vi "KE622x -- Turn Output On And Check For Errors.vi"(0 "Resource In":refnum<visa-resource-name>, 1 "Check For SCPI Errors? (T)":bool=TRUE, 5 "Turn Off Output If Compliance?":bool=TRUE, 11 "error in (no error)":errorcluster, 12 "Compliance Check Delay (500 ms)":u32=500) -> (4 "Resource Out (dupl)":refnum<visa-resource-name>, 6 "Interlock Tripped?":bool, 8 "Compliance?":bool, 15 "error out":errorcluster)   [LabVIEW 2013, in "Keithly user program.lvlib"]
uses:
  Keithly user program.lvlib
  Typedefs/KE622x -- On Off Control.ctl
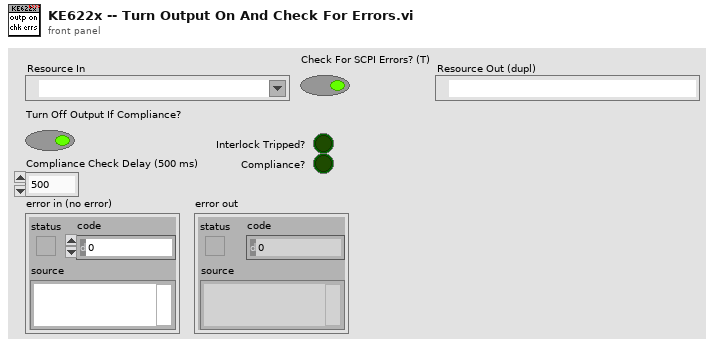
[diagram p1: front panel]
types:
  T1 = typedef "Keithly user program.lvlib/KE622x -- On Off Control.ctl" = enum16{"Off", "On"}
  T2 = typedef "Keithly user program.lvlib/KE622x -- Meas Event Reg State.ctl" = cluster{"B0, ROF:  KE2182A Delta Reading Overflow Event?":bool, "B1, Int:  Interlock OK Event?":bool, "B2, Temp:  Over Temperature Event?":bool, "B3, Comp:  Compliance Event?":bool, "B5, RAV:  Delta Reading Available Event?":bool, "B6, TN:  User Defined Reading Number Stored In Buffer Event?":bool, "B7, BAV:  At Least 2 Readings Stored In Buffer Event?":bool, "B12, BQF:  Buffer Quarter Full Event?":bool, "B8, BHF:  Buffer Half Full Event?":bool, "B13, B3QF:  Buffer 3/4 Full Event?":bool, "B9, BFL:  Buffer Full Event?":bool}
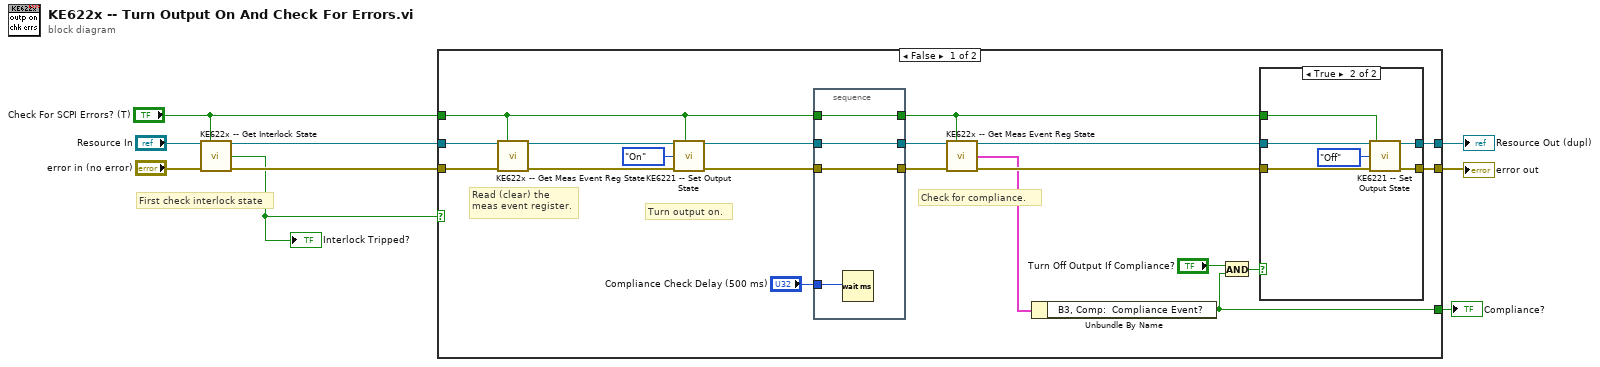
[diagram p0: block diagram]
diagram:
  # "First check interlock state"
  n1 = call "KE622x -- Get Interlock State.vi"("Resource In"="Resource In", "Check For SCPI Errors? (T)"="Check For SCPI Errors? (T)", "error in (no error)"="error in (no error)") -> ("Resource Out (dupl)"=w6:refnum<visa-resource-name>, "Interlock Tripped?"=w2:bool, "error out"=w3:errorcluster)  [unwired: 10 in]
  "Interlock Tripped?" <- w2
  n2 = case shown="False" w2 {
    tunnel: w3 -> [w22 w42]
    tunnel: w6 -> [w23 w43]
    tunnel: "Check For SCPI Errors? (T)" -> [w20 _]
    tunnel: [w27 _] -> w9
    tunnel: [w25 w42] -> w7
    tunnel: [w24 w43] -> w8
    frame False {
      # "Read (clear) the\nmeas event register."
      # "Turn output on."
      # "Check for compliance."
      n3 = call "KE622x -- Get Meas Event Reg State.vi"("VISA Resource In"=w23, "Error Query (T)?"=w20, "error in (no error)"=w22) -> ("VISA Resource Out (dupl)"=w19:refnum<visa-resource-name>, "error out"=w18:errorcluster)  [unwired: 10 in, 1 out]
      n4 = call "KE6221 -- Set Output State.vi"("Resource In"=w19, "Check For SCPI Errors? (T)"=w20, "Output State"=KE622x_--_On_Off_Control."On", "error in (no error)"=w18) -> ("Resource Out (dupl)"=w21:refnum<visa-resource-name>, "error out"=w17:errorcluster)  [unwired: 10 in]
      n5 = stacked-sequence {
        tunnel: "Compliance Check Delay (500 ms)" -> [w41]
        tunnel: w21 -> [w40]
        tunnel: w17 -> [w39]
        tunnel: [w40] -> w16
        tunnel: [w39] -> w13
        tunnel: w20 -> [w38]
        tunnel: [w38] -> w14
        frame #0 {
          n6 = Wait (ms)(milliseconds to wait=w41) -> ()  [unwired: 1 out]
        }
      }
      n7 = call "KE622x -- Get Meas Event Reg State.vi"("VISA Resource In"=w16, "Error Query (T)?"=w14, "error in (no error)"=w13) -> ("VISA Resource Out (dupl)"=w15:refnum<visa-resource-name>, "KE622x Meas Event Reg"=w11:T2, "error out"=w12:errorcluster)  [unwired: 10 in]
      n8 = Unbundle By Name(w11) -> ("B3, Comp:  Compliance Event?"=w27:bool)
      n9 = And(x="Turn Off Output If Compliance?", y=w27) -> (x .and. y?=w26:bool)
      n10 = case shown="True" w26 {
        tunnel: w15 -> [w31 w35]
        tunnel: w12 -> [w30 w34]
        tunnel: w14 -> [_ w33]
        tunnel: [w30 w36] -> w25
        tunnel: [w31 w37] -> w24
        frame False {
        }
        frame True {
          n11 = call "KE6221 -- Set Output State.vi"("Resource In"=w35, "Check For SCPI Errors? (T)"=w33, "Output State"=KE622x_--_On_Off_Control."Off", "error in (no error)"=w34) -> ("Resource Out (dupl)"=w37:refnum<visa-resource-name>, "error out"=w36:errorcluster)  [unwired: 10 in]
        }
      }
    }
    frame True {
    }
  }
  "Resource Out (dupl)" <- w8
  "error out" <- w7
  "Compliance?" <- w9
